vi "f_7_DvDtON.vi"(0 "file path (IN)":path, 1 "Project #":string, 2 "Request #":string, 3 "TEST #":string, 5 "error in (no error)":errorcluster, 6 "VCE":dbl) -> (11 "Dv (V)":dbl, 13 "Dt (ns)":dbl, 14 "file path (OUT)":path, 15 "Dv/Dt (V/us)":dbl, 16 "DONE Dv/Dt ON":bool, 19 "error out":errorcluster)   [LabVIEW 2020]
uses:
  GlobIndSw1.vi
  <vilib>/Waveform/WDTOps.llb/WDT Waveform Duration DBL.vi
  <vilib>/Waveform/WDTOps.llb/WDT Get Waveform Subset DBL.vi
  <vilib>/measure/mamon.llb/Trigger Detection for 1 Channel.vi
  <vilib>/Analysis/NI_AALBase.lvlib
  <vilib>/measure/NI_MAPro.lvlib
panel:
  in  "Decision ?":bool
  out "Dt (us)":dbl
  out "10% Vce":dbl
  out "75% Vce":dbl
  out "Cursor b : Channel 3":dbl
  out "Cursor a : Channel 3":dbl
  out "Waveform Graph":waveform(dbl)[](graph)
  out "ON Region":waveform(dbl)[](graph) caption="DvDt on (V/us)"
  # "Dv/dt(on) = from 75% to 10% of the nominal voltage"
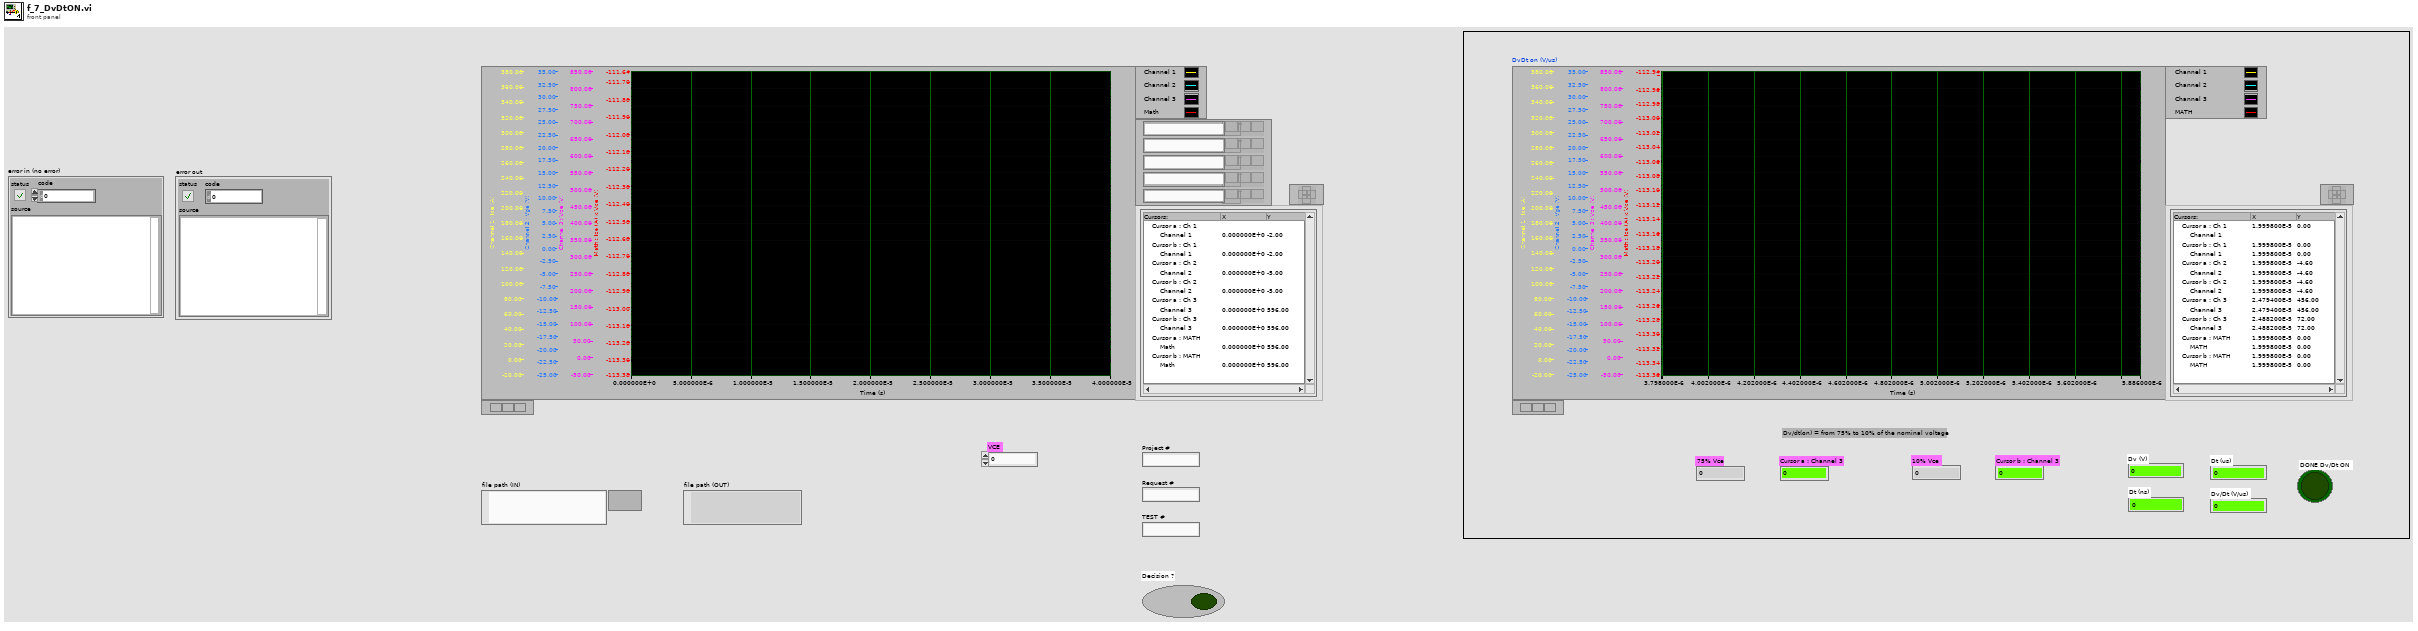
[diagram p1: front panel]
types:
  T1 = enum32{"Invalid", "Standard", "Closed", "Hidden", "Minimized", "Maximized"}
  T2 = typedef "imagedata.ctl" = cluster{"image type":i32, "image depth":i32, "image":u8[], "mask":u8[], "colors":u32[], "Rectangle":cluster{"left":i16, "top":i16, "right":i16, "bottom":i16}}
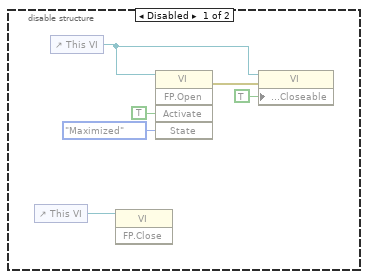
[diagram p2: hidden frame]
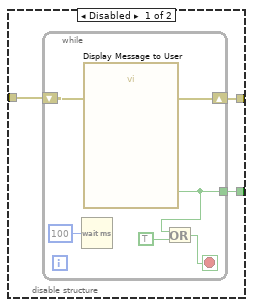
[diagram p3: hidden frame]
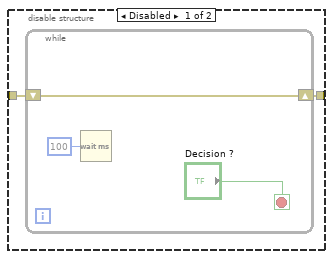
[diagram p8: hidden frame]
diagram:
  w2 = 0.0 ("Dv (V)")
  w3 = errorcluster {"status"=FALSE, "code"=0, "source"=""} ("error out")
  w1 = FALSE ("DONE Tdon")
  w4 = waveform(dbl)[] [] ("Waveform Graph")
  n1 = local write "Cursor a : Channel 3"(w2) -> ()
  n2 = local write "Dv (V)"(w2) -> ()
  n3 = local write "Dt (ns)"(w2) -> ()
  n4 = local write "Dt (us)"(w2) -> ()
  n5 = local write "Dv/Dt (V/us)"(w2) -> ()
  n6 = local write "Cursor b : Channel 3"(w2) -> ()
  n7 = local write "error out"(w3) -> ()
  n8 = local write "error in (no error)"(w3) -> ()
  n9 = local write "DONE Dv/Dt ON"(w1) -> ()
  n10 = local write "Waveform Graph"(w4) -> ()
  n11 = local write "ON Region"(w4) -> ()
  n12 = local write "Decision ?"(w1) -> ()
  n13 = disable-structure shown="Enabled" {
    frame Disabled {
      n14 = control-ref of="This VI"() -> (w11:refnum<vi>)
      n15 = control-ref of="This VI"() -> (w12:refnum<vi>)
      n16 = invoke class="VI" method="FP.Close"(reference=w11) -> ()  [unwired: 2 in, 3 out]
      n17 = invoke class="VI" method="FP.Open"(reference=w12, "Activate"=TRUE ("Activate?"), "State"=T1."Maximized") -> (error in=w15:errorcluster, error out=w13:errorcluster)  [unwired: 1 in, 4 out]
      n18 = property class="VI"(reference=w12, error in=w13, "Front Panel.Closeable"=TRUE ("Front Panel Window:Closeable")) -> ()  [unwired: 2 out]
    }
    frame Enabled {
    }
  }
  n19 = flat-sequence {
    tunnel: [w19] -> w10
    tunnel: ["file path (IN)"] -> w9
    tunnel: [w29] -> w8
    tunnel: [w28] -> w7
    tunnel: w10 -> [w27]
    tunnel: w9 -> [w26]
    tunnel: w8 -> [w286]
    tunnel: [w285] -> w6
    tunnel: [w284] -> w5
    tunnel: w7 -> [w284]
    tunnel: w6 -> [w299]
    tunnel: w5 -> [w300]
    frame #0 {
      n20 = control-ref of="This VI"() -> (w24:refnum<vi>)
      n21 = invoke class="VI" method="FP.Open"(reference=w24, error in="error in (no error)", "Activate"=TRUE ("Activate?"), "State"=T1."Maximized") -> (error out=w25:errorcluster)  [unwired: 1 in, 4 out]
      n22 = property class="VI"(reference=w24, error in=w25, "Front Panel.Closeable"=TRUE ("Front Panel Window:Closeable")) -> (error out=w19:errorcluster)  [unwired: 1 out]
    }
    frame #1 {
      n23 = while {
        tunnel: [w34] -> w28
        shift-right: [w35] -> w29
        shift-left: w27 -> [w33]
        tunnel: w26 -> [w31]
        stop <- w37 stop-if-true
        n24 = flat-sequence {
          tunnel: w33 -> [w72]
          tunnel: [w72] -> w32
          tunnel: w31 -> [w71]
          tunnel: [w71] -> w30
          tunnel: [w94] -> w55
          tunnel: [w84] -> w54
          tunnel: [w74] -> w53
          tunnel: w32 -> [w169]
          tunnel: w30 -> [w163]
          tunnel: w55 -> [w213]
          tunnel: [w223] -> w52
          tunnel: w54 -> [w232]
          tunnel: [w232] -> w51
          tunnel: [w222] -> w50
          tunnel: [w221] -> w49
          tunnel: [w204] -> w48
          tunnel: [w214] -> w47
          tunnel: w53 -> [w206]
          tunnel: w52 -> [w251]
          tunnel: [w250] -> w46
          tunnel: w51 -> [w254]
          tunnel: [w254] -> w45
          tunnel: w50 -> [w253]
          tunnel: [w253] -> w44
          tunnel: w49 -> [w252]
          tunnel: [w252] -> w43
          tunnel: w48 -> [w244]
          tunnel: [w244] -> w42
          tunnel: w47 -> [w245]
          tunnel: [w245] -> w41
          tunnel: w46 -> [w256]
          tunnel: w45 -> [w269]
          tunnel: [w269] -> w40
          tunnel: w44 -> [w263]
          tunnel: w43 -> [w264]
          tunnel: w42 -> [w262]
          tunnel: w41 -> [w261]
          tunnel: [w256] -> w39
          tunnel: w40 -> [w274]
          tunnel: w39 -> [w276]
          tunnel: [w275] -> w38
          tunnel: [w274] -> w34
          frame #0 {
            w69 = 0.0 ("Dv (V)")
            w68 = FALSE ("DONE Tdon")
            w70 = waveform(dbl)[] [] ("Waveform Graph")
            n25 = Wait (ms)(milliseconds to wait=u32 400) -> ()  [unwired: 1 out]
            n26 = local write "Cursor a : Channel 3"(w69) -> ()
            n27 = local write "Dv (V)"(w69) -> ()
            n28 = local write "Dt (ns)"(w69) -> ()
            n29 = local write "Dt (us)"(w69) -> ()
            n30 = local write "Dv/Dt (V/us)"(w69) -> ()
            n31 = local write "Cursor b : Channel 3"(w69) -> ()
            n32 = local write "DONE Dv/Dt ON"(w68) -> ()
            n33 = local write "Decision ?"(w68) -> ()
            n34 = local write "Waveform Graph"(w70) -> ()
            n35 = local write "ON Region"(w70) -> ()
          }
          frame #1 {
            w144 = u16 1 items=["Samples", "Relative Time"] ("start/duration format")
            w155 = u16 1 items=["Samples", "Relative Time"] ("start/duration format")
            w156 = u16 1 items=["Samples", "Relative Time"] ("start/duration format")
            # "Channel 1"
            # "Channel 3"
            # "Channel 2"
            # "dt"
            # "Ch2"
            # "Ch1"
            n36 = call "3_ReadDatatoWaveform.vi"("error in (no error)"=w169, "file path (IN)"=w163) -> ("error out"=w78:errorcluster, "Waveform Graph"=→"Waveform Graph":waveform(dbl)[], "file path (OUT)"=w84:path, "dt"=w164:dbl, "Ch 2 Data"=w161:dbl[], "Ch 3 Data"=w165:dbl[], "Ch 1 Data"=w162:dbl[])  [unwired: 3 in]
            n37 = call <vilib>:"Beep.vi"("use system alert? (T)"=FALSE, "duration (msec)"=u32 200, "frequency (Hz)"=u32 2000) -> ()  [unwired: 9 in]
            n38 = Wait (ms)(milliseconds to wait=u32 400) -> ()  [unwired: 1 out]
            n39 = To Time Stamp(1:0.0 ("number")) -> (0:w166:timestamp)
            n40 = disable-structure shown="Enabled" {
              disable-tunnel: w166 -> [w192 _]
              disable-tunnel: w164 -> [w191 _]
              disable-tunnel: w161 -> [w190 _]
              disable-tunnel: [w189 _] -> w142
              frame Enabled {
                # "Channel 2"
                n41 = Bundle By Name("Y"=w190, "dt"=w191, "t0"=w192) -> (w189:waveform(dbl))  [unwired: 1 in]
              }
              frame Disabled {
              }
            }
            n42 = disable-structure shown="Enabled" {
              disable-tunnel: w166 -> [w188 _]
              disable-tunnel: w164 -> [w187 _]
              disable-tunnel: w162 -> [w186 _]
              disable-tunnel: [w185 _] -> w143
              frame Enabled {
                # "Channel 1"
                n43 = Bundle By Name("Y"=w186, "dt"=w187, "t0"=w188) -> (w185:waveform(dbl))  [unwired: 1 in]
              }
              frame Disabled {
              }
            }
            n44 = disable-structure shown="Enabled" {
              disable-tunnel: w166 -> [w196 _]
              disable-tunnel: w164 -> [w195 _]
              disable-tunnel: w165 -> [w194 _]
              disable-tunnel: [w193 _] -> w141
              disable-tunnel: [w193 _] -> w79
              frame Enabled {
                # "Channel 3"
                n45 = Bundle By Name("Y"=w194, "dt"=w195, "t0"=w196) -> (w193:waveform(dbl))  [unwired: 1 in]
              }
              frame Disabled {
              }
            }
            n46 = disable-structure shown="Enabled" {
              disable-tunnel: w79 -> [w181 _]
              disable-tunnel: w78 -> [w173 _]
              disable-tunnel: [w172 _] -> w75
              disable-tunnel: [w171 _] -> w74
              frame Enabled {
                w175 = u16 1 items=["Samples", "Relative Time"] ("start/duration format")
                # "Channel 3 - Filtered"
                # "Median"
                n47 = global read "GlobIndSw1.vi" "Median Filter Rank"() -> (w170:i32)
                n48 = Unbundle By Name(w181) -> ("Y"=w184:dbl[], "dt"=w182:dbl)
                n49 = call <vilib>:"Median Filter.vi"("right rank"=w170, "left rank"=w170, "X"=w184) -> ("Filtered X"=w183:dbl[])  [unwired: 7 in, 1 out]
                n50 = Bundle By Name("Y"=w183, "dt"=w182) -> (w174:waveform(dbl))  [unwired: 1 in]
                n51 = call-poly <vilib>:"Waveform Duration.vi"("error in (no error)"=w173, "waveform in"=w174) -> ("error out"=w178:errorcluster, "duration"=w180:dbl, "waveform out"=w179:waveform(dbl))  [unwired: 7 in]
                n52 = Divide(x=w180, y=2.0) -> (x/y=w177:dbl)
                n53 = call-poly <vilib>:"Get Waveform Subset.vi"("start/duration format"=w175, "error in (no error)"=w178, "duration"=w177, "start samples/time"=w177, "waveform in"=w179) -> ("error out"=w172:errorcluster, "waveform out"=w171:waveform(dbl))  [unwired: 1 in, 2 out]
              }
              frame Disabled {
              }
            }
            n54 = call-poly <vilib>:"Waveform Duration.vi"("error in (no error)"=w78, "waveform in"=w141) -> ("error out"=w149:errorcluster, "duration"=w146:dbl, "waveform out"=w148:waveform(dbl))  [unwired: 7 in]
            n55 = call-poly <vilib>:"Waveform Duration.vi"("error in (no error)"=w78, "waveform in"=w142) -> ("error out"=w150:errorcluster, "duration"=w153:dbl, "waveform out"=w151:waveform(dbl))  [unwired: 7 in]
            n56 = call-poly <vilib>:"Waveform Duration.vi"("error in (no error)"=w78, "waveform in"=w143) -> ("error out"=w160:errorcluster, "duration"=w157:dbl, "waveform out"=w159:waveform(dbl))  [unwired: 7 in]
            n57 = Divide(x=w146, y=2.0) -> (x/y=w145:dbl)
            n58 = Divide(x=w153, y=2.0) -> (x/y=w154:dbl)
            n59 = Divide(x=w157, y=2.0) -> (x/y=w139:dbl)
            n60 = call-poly <vilib>:"Get Waveform Subset.vi"("start/duration format"=w144, "error in (no error)"=w149, "duration"=w145, "start samples/time"=w145, "waveform in"=w148) -> ("error out"=w76:errorcluster, "waveform out"=w80:waveform(dbl))  [unwired: 1 in, 2 out]
            n61 = call-poly <vilib>:"Get Waveform Subset.vi"("start/duration format"=w155, "error in (no error)"=w150, "duration"=w154, "start samples/time"=w154, "waveform in"=w151) -> ("error out"=w137:errorcluster, "waveform out"=w96:waveform(dbl))  [unwired: 1 in, 2 out]
            n62 = call-poly <vilib>:"Get Waveform Subset.vi"("start/duration format"=w156, "error in (no error)"=w160, "duration"=w139, "start samples/time"=w139, "waveform in"=w159) -> ("error out"=w138:errorcluster, "waveform out"=w95:waveform(dbl))  [unwired: 1 in, 2 out]
            n63 = Build Array(w95, w96, w80, waveform(dbl) {"t0"=timestamp(0 s since 1904-01-01), "dt"=1.0, "Y"=[]} ("element")) -> (→"ON Region":waveform(dbl)[])
            n64 = Merge Errors(w138, w137, w76, w75) -> (w92:errorcluster)
            n65 = property on="ON Region" class="WFGraph (strict)"(error in=w92) -> (error out=w91:errorcluster, "Width"=w90:u32)  [unwired: 1 in, 1 out]
            n66 = property on="ON Region" class="WFGraph (strict)"(error in=w91, "Caption.Justify"=enum16{"Left", "Center", "Right"}."Left" ("Caption.Justification"), "Caption.Width"=w90, "Caption.FontBold"=TRUE ("Caption.Font:Bold"), "Caption.FontColor"=u32 16860 ("Caption.Font:Color"), "Caption.FontSize"=u32 24 ("Caption.Font:Size"), "Caption.Text"="DvDt on (V/us)") -> (error out=w86:errorcluster)  [unwired: 1 in, 1 out]
            n67 = property on="ON Region" class="WFGraph (strict)"(error in=w86, "XScale.Offset"=w139) -> (error out=w120:errorcluster)  [unwired: 1 in, 1 out]
            n68 = property on="ON Region" class="WFGraph (strict)"(error in=w120, "Active Cursor"=u32 0, "Cursor.Cursor X"=0.0 ("Cursor.Cursor Position:Cursor X"), "Cursor.Cursor Y"=0.0 ("Cursor.Cursor Position:Cursor Y"), "Cursor.Visible"=FALSE) -> (error out=w119:errorcluster)  [unwired: 1 in, 1 out]
            n69 = property on="ON Region" class="WFGraph (strict)"(error in=w119, "Active Cursor"=u32 1, "Cursor.Cursor X"=0.0 ("Cursor.Cursor Position:Cursor X"), "Cursor.Cursor Y"=0.0 ("Cursor.Cursor Position:Cursor Y"), "Cursor.Visible"=FALSE) -> (error out=w118:errorcluster)  [unwired: 1 in, 1 out]
            n70 = property on="ON Region" class="WFGraph (strict)"(error in=w118, "Active Cursor"=u32 2, "Cursor.Cursor X"=0.0 ("Cursor.Cursor Position:Cursor X"), "Cursor.Cursor Y"=0.0 ("Cursor.Cursor Position:Cursor Y"), "Cursor.Visible"=FALSE) -> (error out=w117:errorcluster)  [unwired: 1 in, 1 out]
            n71 = property on="ON Region" class="WFGraph (strict)"(error in=w117, "Active Cursor"=u32 3, "Cursor.Cursor X"=0.0 ("Cursor.Cursor Position:Cursor X"), "Cursor.Cursor Y"=0.0 ("Cursor.Cursor Position:Cursor Y"), "Cursor.Visible"=FALSE) -> (error out=w100:errorcluster)  [unwired: 1 in, 1 out]
            n72 = property on="ON Region" class="WFGraph (strict)"(error in=w100, "Active Cursor"=u32 4, "Cursor.Cursor X"=0.0 ("Cursor.Cursor Position:Cursor X"), "Cursor.Cursor Y"=0.0 ("Cursor.Cursor Position:Cursor Y"), "Cursor.Visible"=FALSE) -> (error out=w99:errorcluster)  [unwired: 1 in, 1 out]
            n73 = property on="ON Region" class="WFGraph (strict)"(error in=w99, "Active Cursor"=u32 5, "Cursor.Cursor X"=0.0 ("Cursor.Cursor Position:Cursor X"), "Cursor.Cursor Y"=0.0 ("Cursor.Cursor Position:Cursor Y"), "Cursor.Visible"=FALSE) -> (error out=w98:errorcluster)  [unwired: 1 in, 1 out]
            n74 = property on="ON Region" class="WFGraph (strict)"(error in=w98, "Active Cursor"=u32 6, "Cursor.Cursor X"=0.0 ("Cursor.Cursor Position:Cursor X"), "Cursor.Cursor Y"=0.0 ("Cursor.Cursor Position:Cursor Y"), "Cursor.Visible"=FALSE) -> (error out=w97:errorcluster)  [unwired: 1 in, 1 out]
            n75 = property on="ON Region" class="WFGraph (strict)"(error in=w97, "Active Cursor"=u32 7, "Cursor.Cursor X"=0.0 ("Cursor.Cursor Position:Cursor X"), "Cursor.Cursor Y"=0.0 ("Cursor.Cursor Position:Cursor Y"), "Cursor.Visible"=FALSE) -> (error out=w94:errorcluster)  [unwired: 1 in, 1 out]
          }
          frame #2 {
            w210 = u16 0 items=["Falling Edge", "Rising Edge"] ("trigger slope")
            w211 = u16 1 items=["Index", "Time"] ("location mode")
            w217 = u16 0 items=["Falling Edge", "Rising Edge"] ("trigger slope")
            w218 = u16 1 items=["Index", "Time"] ("location mode")
            # "YPOS"
            # "XPOS"
            # "Cursor a : Channel 3"
            # "Cursor b : Channel 3"
            # "Cursor b : Channel 3"
            # "Cursor a : Channel 3"
            # "Cursor b : Channel 3"
            # "Cursor a : Channel 3"
            # "Cursor b : Channel 3"
            # "Cursor a : Channel 3"
            # "End Time 1st Cursor"
            # "End Time 2nd Cursor"
            # "1st PARAMETER : 75% Vce"
            # "Channel 3"
            # "2nd PARAMETER : 10% Vce"
            # "Channel 3"
            n76 = Divide(x=75.0, y=100.0) -> (x/y=w242:dbl)
            n77 = Wait (ms)(milliseconds to wait=u32 500) -> ()  [unwired: 1 out]
            n78 = call <vilib>:"Beep.vi"("use system alert? (T)"=FALSE, "duration (msec)"=u32 200, "frequency (Hz)"=u32 2000) -> ()  [unwired: 9 in]
            n79 = Multiply(x=w242, y="VCE") -> (x*y=w215:dbl)
            "75% Vce" <- w215
            n80 = Add(x=w215, y=0.2) -> (x+y=w203:dbl)
            n81 = Divide(x=w203, y=10.0) -> (x/y=w201:dbl)
            n82 = call-poly <vilib>:"Basic Level Trigger Detection.vi"("signal in"=w206, "level"=w203, "hysteresis"=w201, "location mode"=w218, "error in (no error)"=w213, "trigger slope"=w217) -> ("trigger location"=w214:dbl, "error out"=w212:errorcluster)  [unwired: 7 in, 1 out]
            n83 = property on="ON Region" class="WFGraph (strict)"(error in=w212, "Active Cursor"=u32 4, "Cursor.Cursor X"=w214, "Cursor.Visible"=TRUE, "Cursor.Cursor Name Visible"=TRUE) -> (error out=w227:errorcluster)  [unwired: 1 in, 1 out]
            n84 = property on="ON Region" class="WFGraph (strict)"(error in=w227, "Active Cursor"=u32 4) -> (error out=w205:errorcluster, "Cursor.Cursor Y"=w222:dbl)  [unwired: 1 in, 1 out]
            "Cursor a : Channel 3" <- w222
            n85 = Divide(x=10.0, y=100.0) -> (x/y=w239:dbl)
            n86 = Multiply(x=w239, y="VCE") -> (x*y=w207:dbl)
            "10% Vce" <- w207
            n87 = Add(x=w207, y=0.2) -> (x+y=w199:dbl)
            n88 = Divide(x=w199, y=10.0) -> (x/y=w198:dbl)
            n89 = call-poly <vilib>:"Basic Level Trigger Detection.vi"("signal in"=w206, "level"=w199, "hysteresis"=w198, "location mode"=w211, "error in (no error)"=w205, "trigger slope"=w210) -> ("trigger location"=w204:dbl, "error out"=w208:errorcluster)  [unwired: 7 in, 1 out]
            n90 = property on="ON Region" class="WFGraph (strict)"(error in=w208, "Active Cursor"=u32 5, "Cursor.Cursor X"=w204, "Cursor.Visible"=TRUE, "Cursor.Cursor Name Visible"=TRUE) -> (error out=w224:errorcluster)  [unwired: 1 in, 1 out]
            n91 = property on="ON Region" class="WFGraph (strict)"(error in=w224, "Active Cursor"=u32 5) -> (error out=w223:errorcluster, "Cursor.Cursor Y"=w221:dbl)  [unwired: 1 in, 1 out]
            "Cursor b : Channel 3" <- w221
          }
          frame #3 {
            # "2nd Cursor"
            # "1st Cursor"
            n92 = Subtract(x=w245, y=1e-06) -> (x-y=w246:dbl)
            n93 = Add(x=w244, y=1e-06) -> (x+y=w247:dbl)
            n94 = property on="ON Region" class="WFGraph (strict)"(error in=w251, "XScale.Minimum"=w246, "XScale.Maximum"=w247) -> (error out=w250:errorcluster)  [unwired: 1 in, 1 out]
            n95 = Wait (ms)(milliseconds to wait=u32 300) -> ()  [unwired: 1 out]
          }
          frame #4 {
            # "us"
            # "ns"
            n96 = Subtract(x=w264, y=w263) -> (x-y=w260:dbl)
            n97 = Subtract(x=w262, y=w261) -> (x-y=w258:dbl)
            n98 = Absolute Value(x=w260) -> (abs(x)=w259:dbl)
            "Dv (V)" <- w259
            n99 = Absolute Value(x=w258) -> (abs(x)=w257:dbl)
            n100 = Multiply(x=w257, y=1000000000.0) -> (x*y=→"Dt (ns)":dbl)
            n101 = Multiply(x=w257, y=1000000.0) -> (x*y=w266:dbl)
            "Dt (us)" <- w266
            n102 = Wait (ms)(milliseconds to wait=u32 300) -> ()  [unwired: 1 out]
            n103 = call <vilib>:"Beep.vi"("use system alert? (T)"=FALSE, "duration (msec)"=u32 200, "frequency (Hz)"=u32 2000) -> ()  [unwired: 9 in]
            n104 = Divide(x=w259, y=w266) -> (x/y=→"Dv/Dt (V/us)":dbl)
          }
          frame #5 {
            n105 = disable-structure shown="Enabled" {
              disable-tunnel: w276 -> [w278 w282]
              disable-tunnel: [w277 w282] -> w275
              frame Disabled {
                n106 = while {
                  shift-right: [w279] -> w277
                  shift-left: w278 -> [w279]
                  stop <- "Decision ?" stop-if-true
                  n107 = Wait (ms)(milliseconds to wait=u32 100) -> ()  [unwired: 1 out]
                }
              }
              frame Enabled {
              }
            }
          }
        }
        n108 = disable-structure shown="Enabled" {
          disable-tunnel: w38 -> [w58 w66]
          disable-tunnel: [w57 TRUE ("NO")] -> w37
          disable-tunnel: [w56 w66] -> w35
          frame Disabled {
            n109 = while {
              tunnel: [w60] -> w57
              shift-right: [w63] -> w56
              shift-left: w58 -> [w64]
              stop <- w62 stop-if-true
              n110 = Wait (ms)(milliseconds to wait=u32 100) -> ()  [unwired: 1 out]
              n111 = call "Display Message to User"("error in (no error)"=w64) -> ("error out"=w63:errorcluster, "NO"=w60:bool)  [unwired: 9 in]
              n112 = Or(x=w60, y=TRUE) -> (x .or. y?=w62:bool)
            }
          }
          frame Enabled {
          }
        }
        n113 = Wait (ms)(milliseconds to wait=u32 100) -> ()  [unwired: 1 out]
      }
    }
    frame #2 {
      w289 = "_"
      n114 = Wait (ms)(milliseconds to wait=u32 300) -> ()  [unwired: 1 out]
      n115 = invoke on="ON Region" class="WFGraph (strict)" method="Get Image"(error in=w286) -> (error out=w292:errorcluster, "image data"=w295:T2)  [unwired: 5 in, 4 out]
      n116 = Concatenate Strings("C:\\Inductive_Switching_Project\\IndSw_Image\\" ("string"), "Project #", w289, "Request #", w289, "TEST #", w289, "DvDton" ("string"), ".png" ("string")) -> (w296:string)
      n117 = String To Path(string=w296) -> (path=w294:path)
      n118 = call <vilib>:"Write PNG File.vi"("error in (no error)"=w292, "image data"=w295, "path to PNG file"=w294) -> ("error out"=w285:errorcluster)  [unwired: 7 in, 1 out]
      "DONE Dv/Dt ON" <- TRUE ("DONE Di/Dt ON")
    }
    frame #3 {
      n119 = disable-structure shown="Enabled" {
        disable-tunnel: w299 -> [w301 _]
        frame Enabled {
          n120 = control-ref of="This VI"() -> (w302:refnum<vi>)
          n121 = invoke class="VI" method="FP.Close"(reference=w302, error in=w301) -> ()  [unwired: 1 in, 3 out]
        }
        frame Disabled {
        }
      }
      "error out" <- w299
      "file path (OUT)" <- w300
    }
  }
